vi "VDH-preLaunchConfig.vi"(10 "preLauch Config":T1, 11 "VDH-VNA_data_handler in":refnum<class "VDH-VNA_data_handler.lvclass">) -> (3 "VDH-VNA_data_handler out":refnum<class "VDH-VNA_data_handler.lvclass">)   [LabVIEW 2020, in "VDH-VNA_data_handler.lvlib" / "VDH-VNA_data_handler.lvclass"]
uses:
  VDH-VNA_data_handler.lvclass
  VDH-preLaunchConfig.ctl
  <vilib>/ActorFramework/Message Enqueuer/Message Enqueuer.lvclass
  VDH-actor_enqueues.ctl
  VDH-VNA_data_handler.lvclass/VDH-VNA_data_handler.ctl
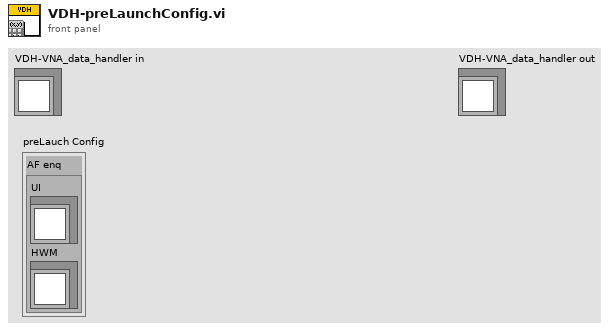
[diagram p1: front panel]
types:
  T1 = typedef "VDH-VNA_data_handler.lvlib/VDH-VNA_data_handler.lvclass/VDH-preLaunchConfig.ctl" = cluster{"AF enq":T2}
  T2 = typedef "VDH-VNA_data_handler.lvlib/VDH-VNA_data_handler.lvclass/VDH-actor_enqueues.ctl" = cluster{"UI":refnum<class "Message Enqueuer.lvclass">, "HWM":refnum<class "Message Enqueuer.lvclass">}
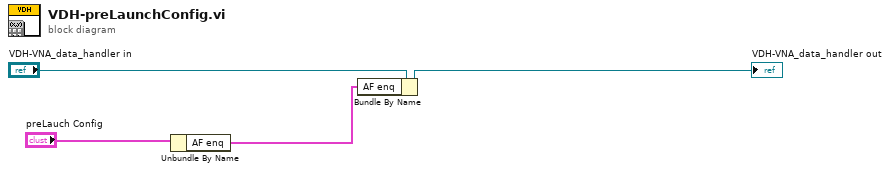
[diagram p0: block diagram]
diagram:
  n1 = Unbundle By Name("preLauch Config") -> ("AF enq"=w1:T2)
  n2 = Bundle By Name(cluster="VDH-VNA_data_handler in", "AF enq"=w1) -> (→"VDH-VNA_data_handler out":refnum<class "VDH-VNA_data_handler.lvclass">)
